vi "Shift Picture.vi"(10 "shift":cluster{"x":i16, "y":i16}, 11 "picture in":picture) -> (3 "picture out":picture)   [LabVIEW 2017]
doc: "Changes position of <b>picture in</b>."
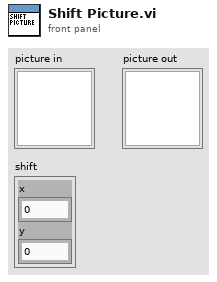
[diagram p1: front panel]
types:
  T1 = typedef "imagedata.ctl" = cluster{"image type":i32, "image depth":i32, "image":u8[], "mask":u8[], "colors":u32[], "Rectangle":cluster{"left":i16, "top":i16, "right":i16, "bottom":i16}}
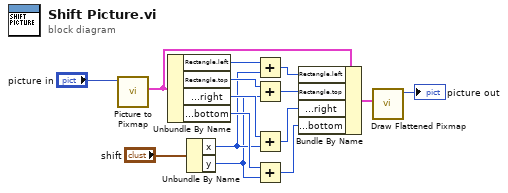
[diagram p0: block diagram]
diagram:
  n1 = call <vilib>:"Picture to Pixmap.vi"("picture"="picture in") -> ("image data"=w5:T1)  [unwired: 9 in, 1 out]
  n2 = Unbundle By Name(w5) -> ("Rectangle.left"=w6:i16, "Rectangle.top"=w7:i16, "Rectangle.right"=w8:i16, "Rectangle.bottom"=w9:i16)
  n3 = Unbundle By Name("shift") -> ("x"=w3:i16, "y"=w2:i16)
  n4 = Add(x=w6, y=w3) -> (x+y=w10:i16)
  n5 = Add(x=w7, y=w2) -> (x+y=w11:i16)
  n6 = Add(x=w8, y=w3) -> (x+y=w12:i16)
  n7 = Add(x=w9, y=w2) -> (x+y=w13:i16)
  n8 = Bundle By Name(cluster=w5, "Rectangle.left"=w10, "Rectangle.top"=w11, "Rectangle.right"=w12, "Rectangle.bottom"=w13) -> (w14:T1)
  n9 = call <vilib>:"Draw Flattened Pixmap.vi"("image data"=w14) -> ("new picture"=→"picture out":picture)  [unwired: 8 in]
